vi "niScope EX Configured Acquisition.vi"() -> ()   [LabVIEW 2021]
doc: "Recommended Input Signal: 100 kHz, 4 Vpp, sine wave\n\nDevices Supported: Refer to NI Example Finder\n\nThis example configures all the oscilloscope's vertical, horizontal, and triggering properties before every acquisition. It allows you to experiment with numerous configurations, including acquisition types and triggering modes, since it supports nearly the entire functionality of NI-SCOPE. However, it is may be more instructive to consult other examples about specific topics such as FlexRes, Random Interleaved Sampling, and Multi-Record to learn more about these features.\n\nMany parameters are included an the front panel of this example. Notice that the \"min sample rate\" is next to the \"actual sample rate,\" and similarly the \"min record length\" is near the \"actual record length.\" The \"min\" values are specified with the Configure Horizontal Timing VI. NI-SCOPE maintains a constant time per record for each acquisition. So when you specify a min sample rate and a min record length, this determines the amount of time the acquisition should take:\n\n time per record = min record length / min sampling rate. \n\nHowever, oscilloscopes support only a certain number of defined sampling rates, so if the value chosen is not a valid rate, it is rounded to the next higher rate, called the actual sample rate. The actual record length is then calculated in order to maintain the time per record. Both of these values are returned in this example so you can investigate the effects of parameter rounding with your oscilloscope. For more information about parameter coercions, see the NI High Speed Digitizers Help.\n\nThe enforce realtime property allows this example to use Random Interleaved Sampling. See the Random Interleaved Sampling example for more details.\n\nKeep in mind that not all digitizers/oscilloscopes support all the features in this example. The NI High Speed Digitizers Help includes a table of supported features for each device."
uses:
  <instrlib>/niScope/Utility/niScope Get Channel Name From String.vi
  <instrlib>/niScope/Configure/Trigger/niScope Configure Trigger Immediate.vi
  <instrlib>/niScope/Configure/Trigger/niScope Configure Trigger Edge.vi
  <instrlib>/niScope/Configure/Trigger/niScope Configure Trigger Digital.vi
  <instrlib>/niScope/Configure/Trigger/niScope Configure Trigger Window.vi
  <instrlib>/niScope/Configure/Trigger/niScope Configure Trigger Hysteresis.vi
  <instrlib>/niScope/Acquire/Fetch/niScope Multi Fetch Cluster.vi
panel:
  in  "Simulate?":bool
  in  "Trigger Type":T1(tab)
  in  "Trigger Source":string(combo)="0"
  in  "Trigger Level":dbl format="%.2f"
  in  "Trigger Slope":i32(ring) items=["Positive", "Negative"]
  in  "Coupling":u16(ring)=1 caption="Trigger Coupling" items=["AC"=0, "DC"=1, "HF Reject"=3, "LF Reject"=4, "AC Plus HF Reject"=1001]
  in  "Trigger Slope":i32(ring) items=["Positive", "Negative"]
  in  "Trigger Source":string(combo)="VAL_PFI_1"
  in  "Coupling":u16(ring)=1 caption="Trigger Coupling" items=["AC"=0, "DC"=1, "HF Reject"=3, "LF Reject"=4, "AC Plus HF Reject"=1001]
  in  "High Level":dbl=0.1 caption="Window High Level" format="%.2f"
  in  "Low Level":dbl=-0.1 caption="Window Low Level" format="%.2f"
  in  "Window Mode":i32(ring) items=["Entering", "Leaving"]
  in  "Trigger Source":string(combo)="0"
  in  "Hysteresis":dbl=0.05 format="%.2f"
  in  "Trigger Source":string(combo)="0"
  in  "Trigger Level":dbl format="%.2f"
  in  "Coupling":u16(ring)=1 caption="Trigger Coupling" items=["AC"=0, "DC"=1, "HF Reject"=3, "LF Reject"=4, "AC Plus HF Reject"=1001]
  in  "Trigger Slope":i32(ring) items=["Positive", "Negative"]
  out "Auto Triggered":bool
  in  "Trigger Modifier":i32(ring)=2 items=["None"=1, "Auto Trigger"=2]
  in  "Vertical Coupling":i32(ring)=1 items=["AC", "DC", "Ground"]
  in  "Stop":bool
  in  "Reference Position":dbl=50.0 caption="Ref Position" format="%.1f"
  in  "Trigger Delay":dbl caption="Trigger Delay (s)" format="%#.4p"
  in  "Maximum Input Frequency":dbl caption="Max. Input Frequency (Hz)" format="%.2f"
  in  "Input Impedance":u32(ring) items=["1 mega ohm"=0, "50 ohms"=2]
  in  "Probe Attenuation":dbl=1.0 format="%.1f"
  in  "Vertical Offset":dbl caption="Vertical Offset (V)" format="%.2p"
  in  "Timeout (s)":dbl=5.0 caption="Timeout(s)" format="%.2f"
  out "Actual Sample Rate":dbl=10000000.0 format="%#.2p"
  out "Actual Record Length":i32=1000
  out "Waveform(s)":T2(graph)
  in  "Min Record Length":i32=1000 caption="Min. Record Length"
  in  "Min Sample Rate":dbl=10000000.0 caption="Min. Sample Rate" step=1000000.0 format="%#.2p"
  in  "Vertical Range":dbl=5.0 caption="Vertical Range (V)" format="%.2f"
  in  "Enforce Realtime":bool=TRUE
  in  "Channel Name":string="0" caption="Channel(s)"
  in  "Resource Name":refnum<k15>="Dev1" caption="Resource Name(s)"
  # "Overview: Demonstrates how to configure vertical, horizontal, and triggering properties and allows you to experiment with numerous configurations, including acquisition types and triggering mode.\nRequirements: NI-SCOPE\nInstructions: \n1. Configure desired acquisition settings.\n2. Run the VI.\n3. Click Stop to stop the VI."
  # "Vertical"
  # "Channel"
  # "Trigger"
  # "Common Trigger Settings"
  # "Horizontal"
  # "Note: When configured for Immediate reference trigger, this example does not configure any additional trigger settings - the acquisition is triggered as soon as possible after being initiated by driver software."
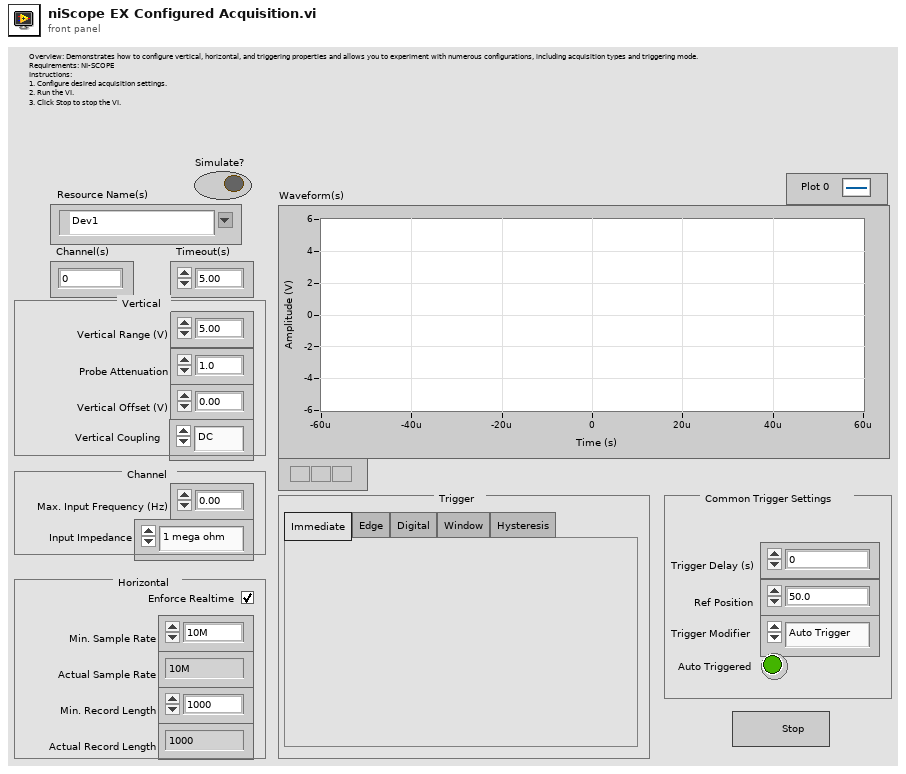
[diagram p1: front panel]
types:
  T1 = enum32{"Immediate", "Edge", "Digital", "Window", "Hysteresis"}
  T2 = cluster{"relativeInitialX":dbl, "xIncrement":dbl, "wfm":dbl[]}[]
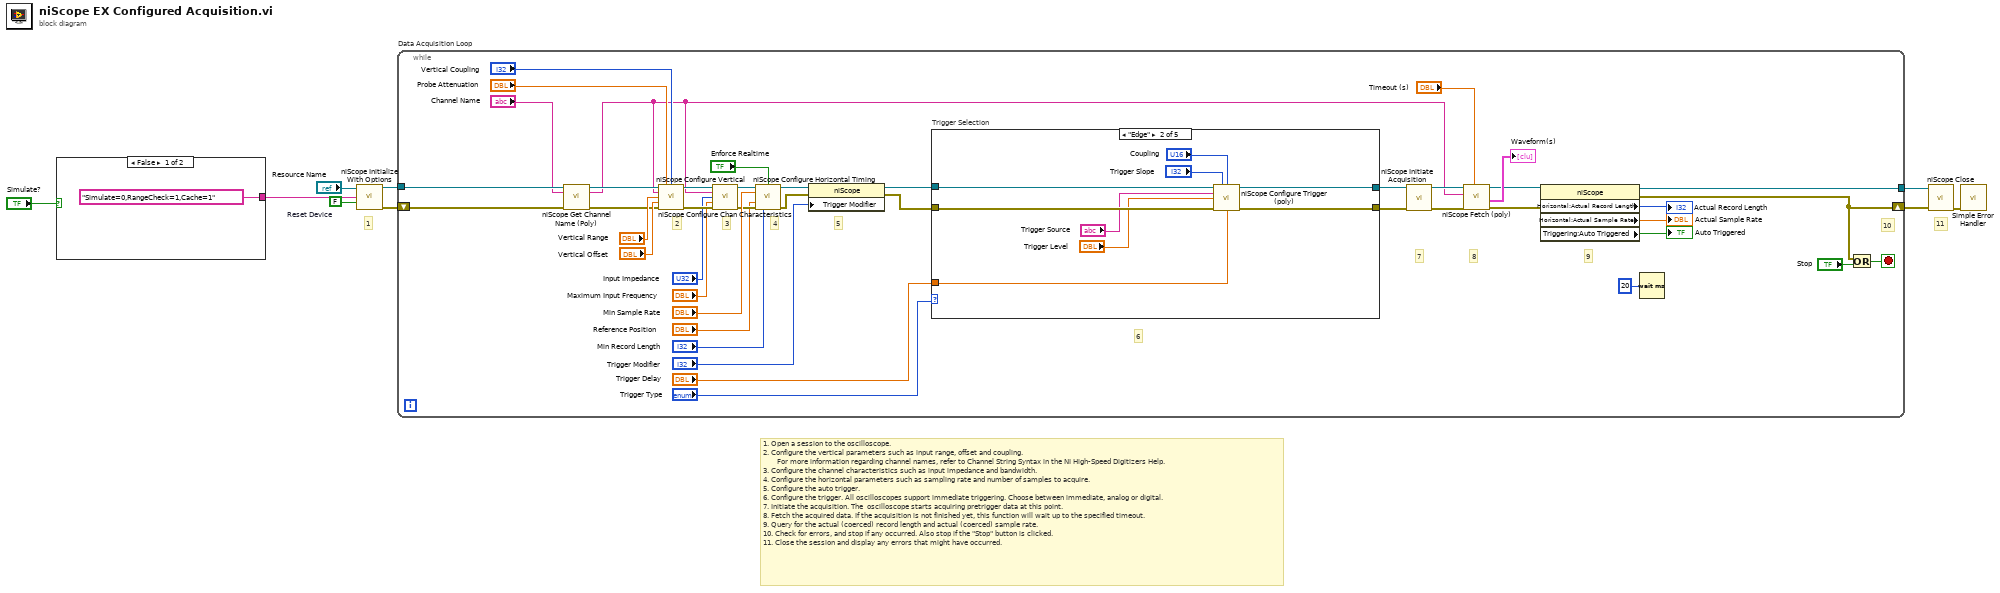
[diagram p0: block diagram]
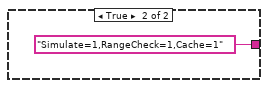
[diagram p2: hidden frame]
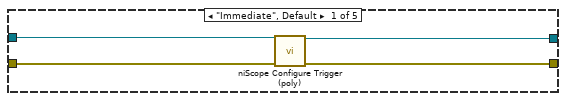
[diagram p3: hidden frame]
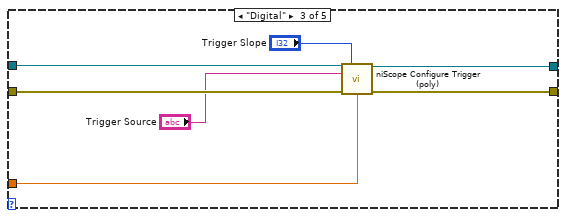
[diagram p4: hidden frame]
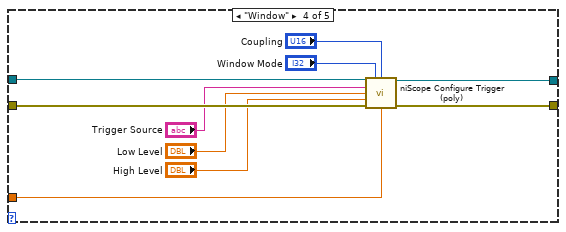
[diagram p5: hidden frame]
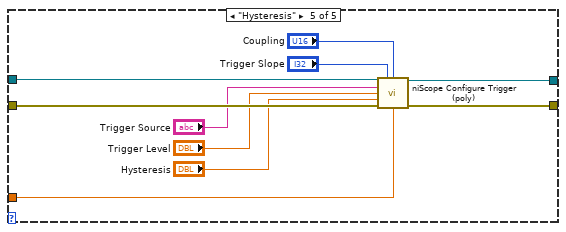
[diagram p6: hidden frame]
diagram:
  w9 = FALSE  # Reset Device
  # "1. Open a session to the oscilloscope.\n2. Configure the vertical parameters such as input range, offset and coupling.\n       For more information regarding channel names, refer to Channel String Syntax in the NI High-Speed Digitizers Help.\n3. Configure the channel characteristics such as input impedance and bandwidth.\n4. Configure the horizontal parameters such as sampling rate and number of samples to acquire.\n5. Configure the auto trigger.\n6. Configure the trigger. All oscilloscopes support immediate triggering. Choose between immediate, analog or digital.\n7. Initiate the acquisition. The  oscilloscope starts acquiring pretrigger data at this point.\n8. Fetch the acquired data. If the acquisition is not finished yet, this function will wait up to the specified timeout.\n9. Query for the actual (coerced) record length and actual (coerced) sample rate.\n10. Check for errors, and stop if any occurred. Also stop if the \"Stop\" button is clicked.\n11. Close the session and display any errors that might have occurred."
  # "11"
  # "1"
  n1 = case shown="False" "Simulate?" {
    tunnel: ["Simulate=0,RangeCheck=1,Cache=1" ("option string") "Simulate=1,RangeCheck=1,Cache=1" ("option string")] -> w1
    frame False {
    }
    frame True {
    }
  }
  n2 = call <instrlib>:"niScope Initialize With Options.vi"("resource name"="Resource Name", "option string"=w1, "reset device"=w9) -> ("instrument handle"=w6:refnum<k15>, "error out"=w3:errorcluster)  [unwired: 11 in]
  n3 = while "Data Acquisition Loop" {
    tunnel: [w24] -> w7
    tunnel: w6 -> [w17]
    shift-right: [w18] -> w5
    shift-left: w3 -> [w14]
    stop <- w38 stop-if-true
    # "5"
    # "2"
    # "3"
    # "4"
    # "6"
    # "7"
    # "8"
    # "9"
    # "10"
    n4 = call-poly <instrlib>:"niScope Get Channel Name (Poly).vi"("instrument handle"=w17, "index"="Channel Name", "error in"=w14) -> ("instrument handle out"=w16:refnum<k15>, "channel name"=w12:string, "error out"=w15:errorcluster)  [unwired: 10 in]
    n5 = call <instrlib>:"niScope Configure Vertical.vi"("instrument handle"=w16, "probe attenuation"="Probe Attenuation", "vertical coupling"="Vertical Coupling", "channels"=w12, "vertical range"="Vertical Range", "vertical offset"="Vertical Offset", "error in"=w15) -> ("instrument handle out"=w51:refnum<k15>, "error out"=w50:errorcluster)  [unwired: 7 in]
    n6 = call <instrlib>:"niScope Configure Chan Characteristics.vi"("instrument handle"=w51, "channels"=w12, "input impedance"="Input Impedance", "maximum input frequency"="Maximum Input Frequency", "error in"=w50) -> ("instrument handle out"=w48:refnum<k15>, "error out"=w49:errorcluster)  [unwired: 9 in]
    n7 = call <instrlib>:"niScope Configure Horizontal Timing.vi"("instrument handle"=w48, "enforce realtime"="Enforce Realtime", "min sample rate"="Min Sample Rate", "reference position"="Reference Position", "error in"=w49, "min record length"="Min Record Length") -> ("instrument handle out"=w31:refnum<k15>, "error out"=w30:errorcluster)  [unwired: 8 in]
    n8 = property on="Property Node" class="niScope"(reference=w31, error in=w30, "Trigger Modifier"="Trigger Modifier") -> (reference out=w28:refnum<k15>, error out=w29:errorcluster)
    n9 = case "Trigger Selection" shown="\"Edge\"" "Trigger Type" {
      tunnel: w29 -> [w58 w67 w74 w84 w94]
      tunnel: [w55 w63 w70 w80 w90] -> w34
      tunnel: w28 -> [w57 w66 w73 w83 w93]
      tunnel: [w56 w64 w71 w81 w92] -> w37
      tunnel: "Trigger Delay" -> [_ w65 w72 w82 w91]
      frame "Immediate", Default {
        n10 = call-poly <instrlib>:"niScope Configure Trigger (poly).vi"("instrument handle"=w57, "error in"=w58) -> ("instrument handle out"=w56:refnum<k15>, "error out"=w55:errorcluster)  [unwired: 12 in]
      }
      frame "Edge" {
        n11 = call-poly <instrlib>:"niScope Configure Trigger (poly).vi"("instrument handle"=w66, "trigger slope"="Trigger Slope", "trigger coupling"="Coupling", "trigger source"="Trigger Source", "trigger level"="Trigger Level", "error in"=w67, "trigger delay"=w65) -> ("instrument handle out"=w64:refnum<k15>, "error out"=w63:errorcluster)  [unwired: 7 in]
      }
      frame "Digital" {
        n12 = call-poly <instrlib>:"niScope Configure Trigger (poly).vi"("instrument handle"=w73, "trigger slope"="Trigger Slope", "trigger source"="Trigger Source", "error in"=w74, "trigger delay"=w72) -> ("instrument handle out"=w71:refnum<k15>, "error out"=w70:errorcluster)  [unwired: 9 in]
      }
      frame "Window" {
        n13 = call-poly <instrlib>:"niScope Configure Trigger (poly).vi"("instrument handle"=w83, "trigger window mode"="Window Mode", "trigger coupling"="Coupling", "trigger source"="Trigger Source", "low level"="Low Level", "high level"="High Level", "error in"=w84, "trigger delay"=w82) -> ("instrument handle out"=w81:refnum<k15>, "error out"=w80:errorcluster)  [unwired: 6 in]
      }
      frame "Hysteresis" {
        n14 = call-poly <instrlib>:"niScope Configure Trigger (poly).vi"("instrument handle"=w93, "trigger slope"="Trigger Slope", "trigger coupling"="Coupling", "trigger source"="Trigger Source", "trigger level"="Trigger Level", "hysteresis"="Hysteresis", "error in"=w94, "trigger delay"=w91) -> ("instrument handle out"=w92:refnum<k15>, "error out"=w90:errorcluster)  [unwired: 6 in]
      }
    }
    n15 = call <instrlib>:"niScope Initiate Acquisition.vi"("instrument handle"=w37, "error in"=w34) -> ("instrument handle out"=w36:refnum<k15>, "error out"=w35:errorcluster)  [unwired: 12 in]
    n16 = call-poly <instrlib>:"niScope Fetch (poly).vi"("timeout"="Timeout (s)", "error in"=w35, "channels"=w12, "instrument handle"=w36) -> ("error out"=w25:errorcluster, "waveform"=→"Waveform(s)":T2, "instrument handle out"=w26:refnum<k15>)  [unwired: 4 in, 1 out]
    n17 = property class="niScope"(reference=w26, error in=w25) -> (reference out=w24:refnum<k15>, error out=w18:errorcluster, "Horizontal:Actual Record Length"=→"Actual Record Length":i32, "Horizontal:Actual Sample Rate"=→"Actual Sample Rate":dbl, "Triggering:Auto Triggered"=→"Auto Triggered":bool)
    n18 = Wait (ms)(milliseconds to wait=u32 20) -> ()  [unwired: 1 out]
    n19 = Or(x=w18, y="Stop") -> (x .or. y?=w38:bool)
  }
  n20 = call <instrlib>:"niScope Close.vi"("instrument handle"=w7, "error in"=w5) -> ("error out"=w8:errorcluster)  [unwired: 13 in]
  n21 = call <vilib>:"Simple Error Handler.vi"("error in (no error)"=w8) -> ()  [unwired: 4 in, 5 out]
